vi "Window-Time series confirm.vi"(8 "error in (no error)":errorcluster) -> (0 "error out":errorcluster, 1 "Cancelled (Left button pressed)":bool, 3 "Panel closed":bool)   [LabVIEW 2020]
doc: "Use this template to create a dialog box with event handling."
uses:
  <vilib>/Utility/miscctls.llb/LVPointTypeDef.ctl
  Global Variables/General Globals.vi
panel:
  in  "Left Button":bool
  in  "Rigth Button":bool
  out "Message":string="Note:\nTime series recording is enabled."
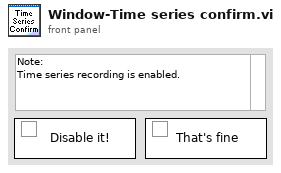
[diagram p1: front panel]
types:
  T1 = typedef "LVPointTypeDef.ctl" = cluster{"Horizontal":i16, "Vertical":i16}
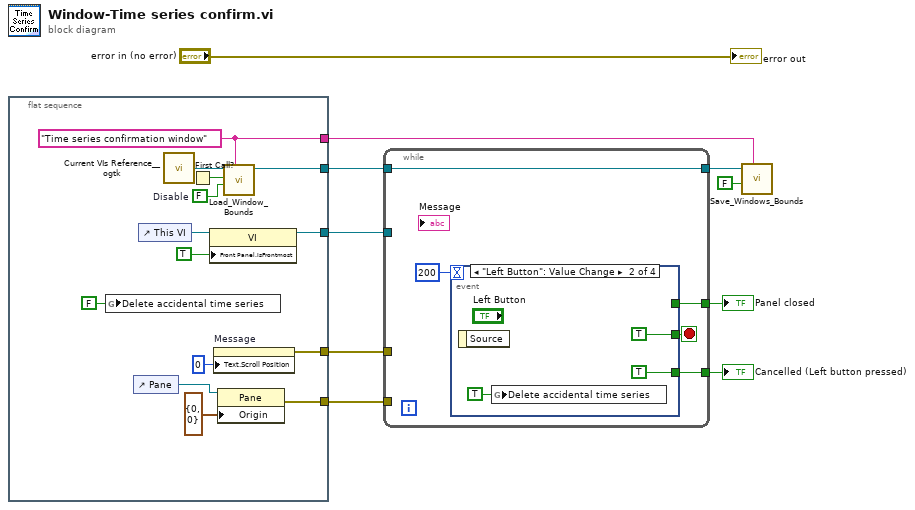
[diagram p0: block diagram]
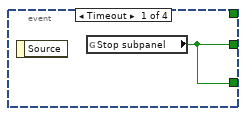
[diagram p2: hidden frame]
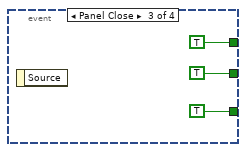
[diagram p3: hidden frame]
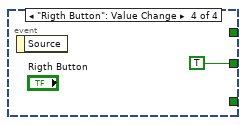
[diagram p4: hidden frame]
diagram:
  n1 = flat-sequence {
    tunnel: [w23] -> w10
    tunnel: [w20] -> w9
    tunnel: [w18] -> w8
    tunnel: [w13] -> w6
    tunnel: [w12] -> w4
    frame #0 {
      w14 = FALSE  # Disable
      w13 = "Time series confirmation window" ("Window Name (i.e. Key)")
      n2 = global write "General Globals.vi" "Delete accidental time series"(FALSE ("Delete accidental time series")) -> ()
      n3 = control-ref of="Pane"() -> (w17:refnum<vi>)
      n4 = control-ref of="This VI"() -> (w21:refnum<vi>)
      n5 = call <userlib>:"Current VIs Reference__ogtk.vi"() -> ("Current VI's reference"=w16:refnum<vi>)  [unwired: 5 in]
      n6 = First Call?() -> (First Call?: T/F=w15:bool)
      n7 = property on="Property Node" class="VI"(reference=w21, "Front Panel.IsFrontmost"=TRUE ("Front Panel Window:Is Frontmost")) -> (reference out=w20:refnum<vi>)  [unwired: 1 in, 1 out]
      n8 = property on="Message" class="Str"("Text.Scroll Position"=u32 0) -> (error out=w23:errorcluster)  [unwired: 2 in, 1 out]
      n9 = property class="Pane"(reference=w17, "Origin"=T1 {"Horizontal"=0, "Vertical"=0}) -> (error out=w18:errorcluster)  [unwired: 1 in, 1 out]
      n10 = call "Load_Window_Bounds.vi"("Window Name (i.e. Key)"=w13, "Disable"=w14, "First Call"=w15, "Window VI's Ref"=w16) -> ("reference out"=w12:refnum<vi>)  [unwired: 4 in, 3 out]
    }
  }
  n11 = while {
    tunnel: w10 -> [_]
    tunnel: w8 -> [_]
    tunnel: w9 -> [_]
    tunnel: [w27] -> w7
    tunnel: w4 -> [w26]
    tunnel: [w26] -> w3
    tunnel: [w25] -> w1
    stop <- w29 stop-if-true
    n12 = event shown="[1] \"Left Button\": Value Change" {
      selector: _ -> [_ _ _ _]
      dyn-events: _ -> [_ _ _ _]
      timeout: 200 -> [_ _ _ _]
      tunnel: [w30 TRUE ("Stop?") TRUE ("Stop?") TRUE ("Stop?")] -> w29
      tunnel: [w30 TRUE ("Stop subpanel") TRUE ("Stop subpanel") _] -> w27
      tunnel: [_ _ TRUE ("Stop subpanel") _] -> w25
      event Timeout {
        n13 = event-data() -> ()  [unwired: 1 in, 1 out]
        n14 = global read "General Globals.vi" "Stop subpanel"() -> (w30:bool)
      }
      event "Left Button": Value Change {
        n15 = event-data() -> ()  [unwired: 1 in, 1 out]
        n16 = global write "General Globals.vi" "Delete accidental time series"(TRUE ("Delete accidental time series")) -> ()
      }
      event Panel Close {
        n17 = event-data() -> ()  [unwired: 1 in, 1 out]
      }
      event "Rigth Button": Value Change {
        n18 = event-data() -> ()  [unwired: 1 in, 1 out]
      }
    }
  }
  "Cancelled (Left button pressed)" <- w7
  "Panel closed" <- w1
  n19 = call "Save_Windows_Bounds.vi"("Window Name (i.e. Key)"=w6, "Front Panel Window:Open"=FALSE, "Window VI's Ref"=w3) -> ()  [unwired: 8 in, 1 out]
  "error out" <- "error in (no error)"
